vi "WriteLogFile.vi"(0 "Path to File":path=path "G:/Développement de Programmes/Programmes/octo-labview/Automatisation Manip Gaz/data/data.dat", 1 "Shot Num":i32, 5 "Pulse Energy fs":dbl, 7 "Pulse Duration fs":dbl, 9 "Pressure reading bar-a":dbl, 11 "Pressure reading mA":dbl, 12 "Comments":string, 13 "Overwrite":bool) -> (6 "Message":string, 8 "Success?":i32)   [LabVIEW 2013]
uses:
  <vilib>/regexp/Match Regular Expression.xnode
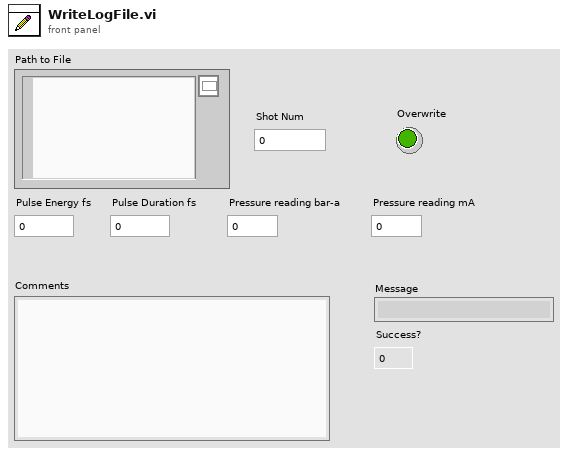
[diagram p1: front panel]
types:
  T1 = enum16{"open", "replace", "create", "open or create", "replace or create", "replace or create with confirmation"}
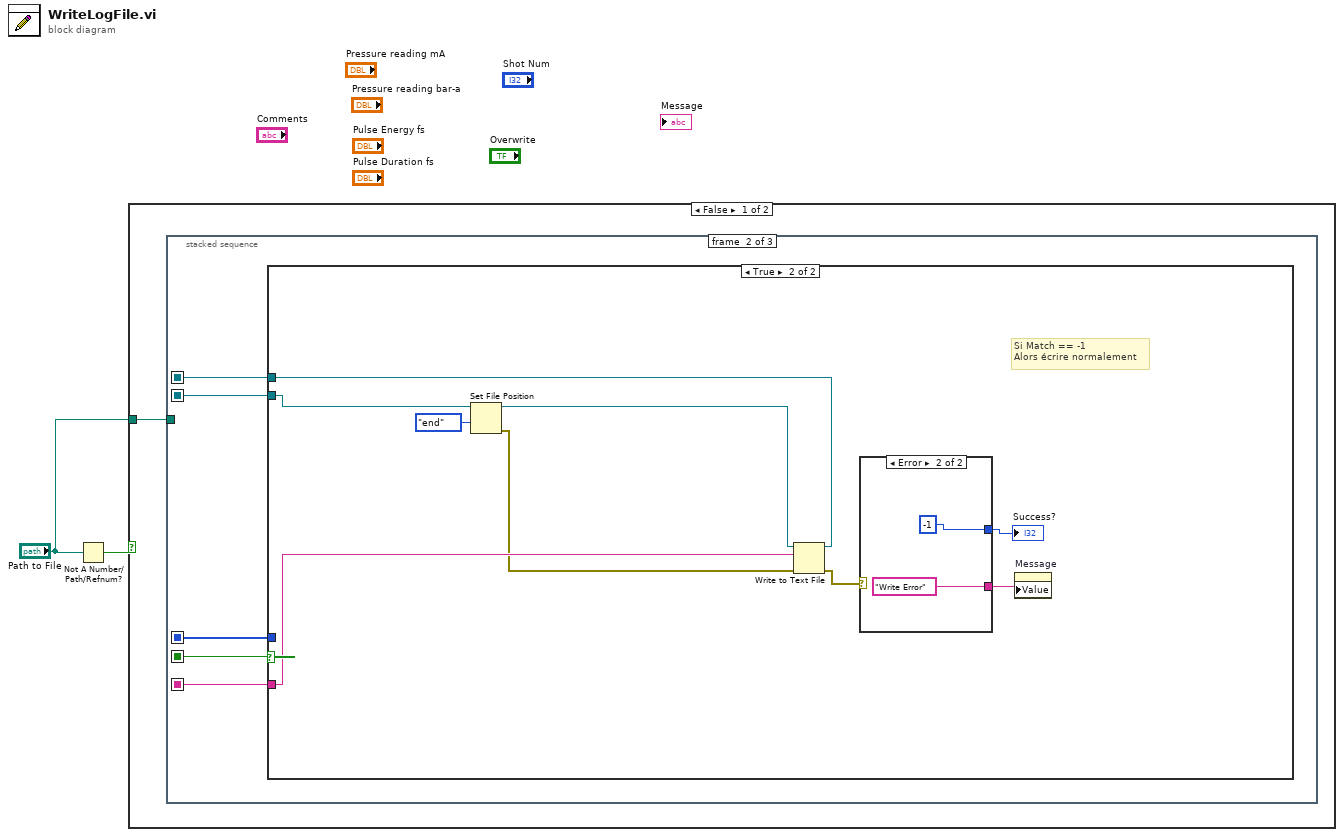
[diagram p0: block diagram]
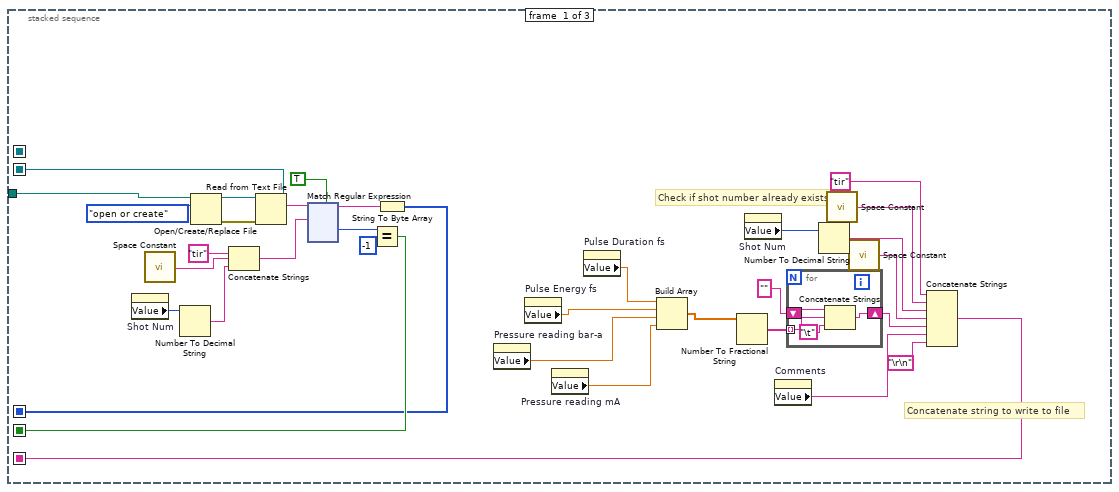
[diagram p2: hidden frame]
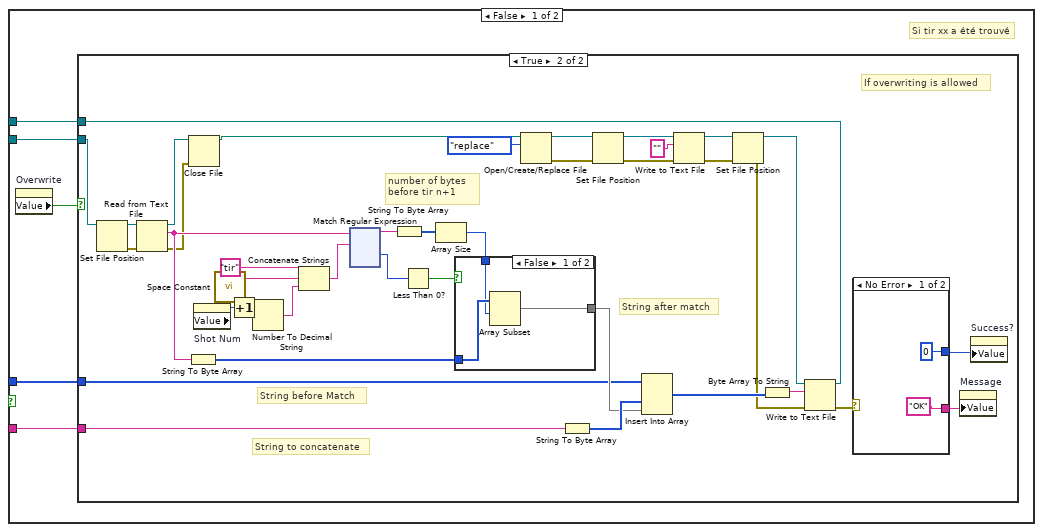
[diagram p3: hidden frame]
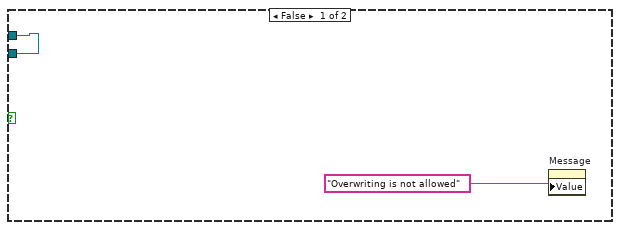
[diagram p4: hidden frame]
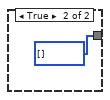
[diagram p5: hidden frame]
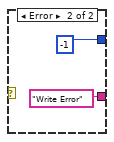
[diagram p6: hidden frame]
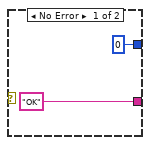
[diagram p7: hidden frame]
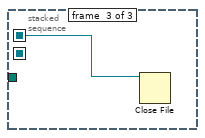
[diagram p8: hidden frame]
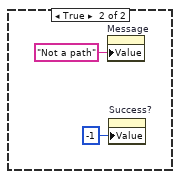
[diagram p9: hidden frame]
diagram:
  n1 = Not A Number/Path/Refnum?(number/path/refnum="Path to File") -> (NaN/Path/Refnum?=w2:bool)
  n2 = case shown="False" w2 {
    tunnel: "Path to File" -> [w3 _]
    frame False {
      n3 = stacked-sequence {
        seq-local: [w26 _ _] -> [_ w158 _]
        seq-local: [_ w157 _] -> [_ _ w341]
        seq-local: [w23 _ _] -> [_ w159 _]
        seq-local: [w20 _ _] -> [_ w156 _]
        seq-local: [w4 _ _] -> [_ w155 _]
        tunnel: w3 -> [w27 _ _]
        frame #0 {
          # "Concatenate string to write to file"
          # "Check if shot number already exists"
          n4 = property on="Shot Num" class="DigNum (strict)"() -> ("Value"=w36:i32)  [unwired: 2 in, 2 out]
          n5 = call <vilib>:"Space Constant.vi"() -> ("String"=w24:string)
          n6 = Number To Decimal String(number=w36) -> (decimal integer string=w25:string)  [unwired: 1 in]
          n7 = Open/Create/Replace File(file path (use dialog)=w27, operation (0:open)=T1."open or create") -> (refnum out=w30:refnum<file>, error out=w29:errorcluster)  [unwired: 4 in, 1 out]
          n8 = Concatenate Strings("tir", w24, w25) -> (w33:string)
          n9 = Read from Text File(file (use dialog)=w30, error in=w29) -> (refnum out=w26:refnum<file>, text=w34:string)  [unwired: 2 in, 2 out]
          n10 = xnode "Match Regular Expression"("input string"=w34, "regular expression"=w33, "multiline? (F)"=TRUE) -> ("before match"=w21:string, "offset past match"=w22:i32)  [unwired: 3 in, 3 out]
          n11 = Equal?(x=w22, y=-1) -> (x = y?=w23:bool)
          n12 = String To Byte Array(string=w21) -> (unsigned byte array=w20:u8[])
          n13 = property on="Pressure reading bar-a" class="DigNum (strict)"() -> ("Value"=w17:dbl)  [unwired: 2 in, 2 out]
          n14 = property on="Pulse Energy fs" class="DigNum (strict)"() -> ("Value"=w18:dbl)  [unwired: 2 in, 2 out]
          n15 = property on="Pressure reading mA" class="DigNum (strict)"() -> ("Value"=w16:dbl)  [unwired: 2 in, 2 out]
          n16 = property on="Pulse Duration fs" class="DigNum (strict)"() -> ("Value"=w19:dbl)  [unwired: 2 in, 2 out]
          n17 = Build Array(w19, w18, w17, w16) -> (w7:dbl[])
          n18 = Number To Fractional String(number=w7) -> (F-format string=w15:string[])  [unwired: 3 in]
          n19 = property on="Shot Num" class="DigNum (strict)"() -> ("Value"=w6:i32)  [unwired: 2 in, 2 out]
          n20 = property on="Comments" class="Str"() -> ("Value"=w8:string)  [unwired: 2 in, 2 out]
          n21 = for {
            tunnel: w15 -> [w40] mode=indexing
            shift-right: [w39] -> w13
            shift-left: "" ("string") -> [w38]
            n22 = Concatenate Strings(w38, w40, "\t") -> (w39:string)
          }
          n23 = Number To Decimal String(number=w6) -> (decimal integer string=w10:string)  [unwired: 1 in]
          n24 = call <vilib>:"Space Constant.vi"() -> ("String"=w9:string)
          n25 = call <vilib>:"Space Constant.vi"() -> ("String"=w11:string)
          n26 = Concatenate Strings("tir" ("string"), w9, w10, w11, w13, w8, "\r\n") -> (w4:string)
        }
        frame #1 {
          n27 = case shown="True" w159 {
            tunnel: w158 -> [w164 w331]
            tunnel: [w163 w334] -> w157
            tunnel: w156 -> [w162 _]
            tunnel: w155 -> [w161 w332]
            frame False {
              # "Si tir xx a été trouvé"
              n28 = property on="Overwrite" class="Bool (strict)"() -> ("Value"=w160:bool)  [unwired: 2 in, 2 out]
              n29 = case shown="True" w160 {
                tunnel: w164 -> [w166 w184]
                tunnel: [w166 w205] -> w163
                tunnel: w162 -> [_ w186]
                tunnel: w161 -> [_ w169]
                frame False {
                  n30 = property on="Message" class="Str"("Value"="Overwriting is not allowed" ("Message")) -> ()  [unwired: 2 in, 2 out]
                }
                frame True {
                  # "String after match"
                  # "String to concatenate"
                  # "String before Match"
                  # "number of bytes \nbefore tir n+1"
                  # "If overwriting is allowed"
                  n31 = Set File Position(refnum=w184) -> (refnum out=w185:refnum<file>, error out=w183:errorcluster)  [unwired: 3 in]
                  n32 = Read from Text File(file (use dialog)=w185, error in=w183) -> (refnum out=w174:refnum<file>, text=w196:string, error out=w168:errorcluster)  [unwired: 2 in, 1 out]
                  n33 = String To Byte Array(string=w196) -> (unsigned byte array=w195:u8[])
                  n34 = Close File(refnum=w174, error in=w168) -> (path=w173:path)  [unwired: 1 out]
                  n35 = property on="Shot Num" class="DigNum (strict)"() -> ("Value"=w200:i32)  [unwired: 2 in, 2 out]
                  n36 = call <vilib>:"Space Constant.vi"() -> ("String"=w202:string)
                  n37 = Increment(x=w200) -> (x+1=w201:i32)
                  n38 = Number To Decimal String(number=w201) -> (decimal integer string=w203:string)  [unwired: 1 in]
                  n39 = Concatenate Strings("tir", w202, w203) -> (w199:string)
                  n40 = xnode "Match Regular Expression"("input string"=w196, "regular expression"=w199) -> ("before match"=w197:string, "offset past match"=w182:i32)  [unwired: 4 in, 3 out]
                  n41 = String To Byte Array(string=w197) -> (unsigned byte array=w198:u8[])
                  n42 = Less Than 0?(x=w182) -> (x < 0?=w181:bool)
                  n43 = Array Size(array=w198) -> (size(s)=w194:i32)
                  n44 = case shown="False" w181 {
                    tunnel: w195 -> [w208 _]
                    tunnel: w194 -> [w207 _]
                    tunnel: [w206 u8[] []] -> w189
                    frame False {
                      n45 = Array Subset(array=w208, index=w207) -> (w206:u8[])  [unwired: 1 in]
                    }
                    frame True {
                    }
                  }
                  n46 = Open/Create/Replace File(file path (use dialog)=w173, operation (0:open)=T1."replace") -> (refnum out=w171:refnum<file>, error out=w170:errorcluster)  [unwired: 4 in, 1 out]
                  n47 = String To Byte Array(string=w169) -> (unsigned byte array=w190:u8[])
                  n48 = Set File Position(refnum=w171, error in=w170) -> (refnum out=w180:refnum<file>, error out=w178:errorcluster)  [unwired: 2 in]
                  n49 = Insert Into Array(array=w186, new element #1=w190, new element #2=w189) -> (w188:u8[])  [unwired: 1 in]
                  n50 = Write to Text File(file (use dialog)=w180, text="", error in=w178) -> (refnum out=w177:refnum<file>, error out=w175:errorcluster)  [unwired: 1 in, 1 out]
                  n51 = Set File Position(refnum=w177, error in=w175) -> (refnum out=w176:refnum<file>, error out=w167:errorcluster)  [unwired: 2 in]
                  n52 = Byte Array To String(unsigned byte array=w188) -> (string=w187:string)
                  n53 = Write to Text File(file (use dialog)=w176, text=w187, error in=w167) -> (refnum out=w205:refnum<file>, error out=w192:errorcluster)  [unwired: 1 in, 1 out]
                  n54 = case shown="No Error" w192 {
                    tunnel: ["OK" ("Message") "Write Error" ("Message")] -> w193
                    tunnel: [0 ("Success?") -1 ("Success?")] -> w191
                    frame No Error {
                    }
                    frame Error {
                    }
                  }
                  n55 = property on="Message" class="Str"("Value"=w193) -> ()  [unwired: 2 in, 2 out]
                  n56 = property on="Success?" class="DigNum (strict)"("Value"=w191) -> ()  [unwired: 2 in, 2 out]
                }
              }
            }
            frame True {
              # "Si Match == -1\nAlors écrire normalement"
              n57 = Set File Position(refnum=w331, from (0:start)=enum16{"start", "end", "current"}."end") -> (refnum out=w330:refnum<file>, error out=w329:errorcluster)  [unwired: 2 in]
              n58 = Write to Text File(file (use dialog)=w330, text=w332, error in=w329) -> (refnum out=w334:refnum<file>, error out=w336:errorcluster)  [unwired: 1 in, 1 out]
              n59 = case shown="Error" w336 {
                tunnel: ["OK" ("Message") "Write Error" ("Message")] -> w335
                tunnel: [0 ("Success?") -1 ("Success?")] -> w333
                frame No Error {
                }
                frame Error {
                }
              }
              "Success?" <- w333
              n60 = property on="Message" class="Str"("Value"=w335) -> ()  [unwired: 2 in, 2 out]
            }
          }
        }
        frame #2 {
          n61 = Close File(refnum=w341) -> ()  [unwired: 1 in, 2 out]
        }
      }
    }
    frame True {
      n62 = property on="Message" class="Str"("Value"="Not a path" ("Message")) -> ()  [unwired: 2 in, 2 out]
      n63 = property on="Success?" class="DigNum (strict)"("Value"=-1 ("Success?")) -> ()  [unwired: 2 in, 2 out]
    }
  }
